vi "Calculate spot profile.vi"() -> ()   [LabVIEW 2012]
uses:
  <vilib>/Utility/file.llb/Write To Spreadsheet File (DBL).vi
panel:
  in  "Intensity":bool
  in  "log":bool
  in  "Save":bool
  in  "N spots":i32=2
  in  "xlog":dbl=2.0
  in  "stop 2":bool
  in  "Minimum":dbl(slide)=-3.5369774919614088 scale=-100.0..100.0
  in  "Maximum mult":dbl(slide)=0.9919614147909966 scale=0.1..2.0
  in  "stop":bool
  out "Spot profile":dbl[][](graph)
  out "Amplitudes/weights":sgl[][](graph)
  in  "I":sgl[](array[numeric])=[7.0, 7.0, 7.0, 7.0, 7.0, 7.0, 10.0, 10.0, 10.0, 10.0, 10.0, 10.0, 10.0, 10.0, 10.0, 10.0, 10.0, 10.0, 10.0, 10.0, 10.0]
  in  "xz-plane":bool=TRUE
  in  "step":sgl=1.0
  in  "N points":i32=512
  in  "Spot to display":i32
  in  "N_iterations":i32=100
  in  "x":sgl[](array[numeric])=[0.0, 40.0, -40.0, 10.0, 20.0, 30.0] format="%#_12g"
  in  "y":sgl[](array[numeric])=[0.0, 0.0, 0.0, 0.0, 0.0, 0.0, 0.0, 0.0, 0.0, 0.0, 0.0, 0.0, 0.0, 0.0, 0.0, 0.0, 0.0, 0.0, 0.0, 0.0, 0.0]
  in  "z":sgl[](array[numeric])=[0.0, 20.0, 20.0, -14.0, 0.0, 30.0, 0.0, 0.0, 0.0, 0.0, 0.0, 0.0, 0.0, 0.0, 0.0, 0.0, 0.0, 0.0, 0.0, 0.0, 0.0]
  in  "method":i32(ring)=1 items=["Lenses & gratings", "GS Fresnel", "GS FFT (2D)"]
  out "Generated Hologram":u8[][](graph)
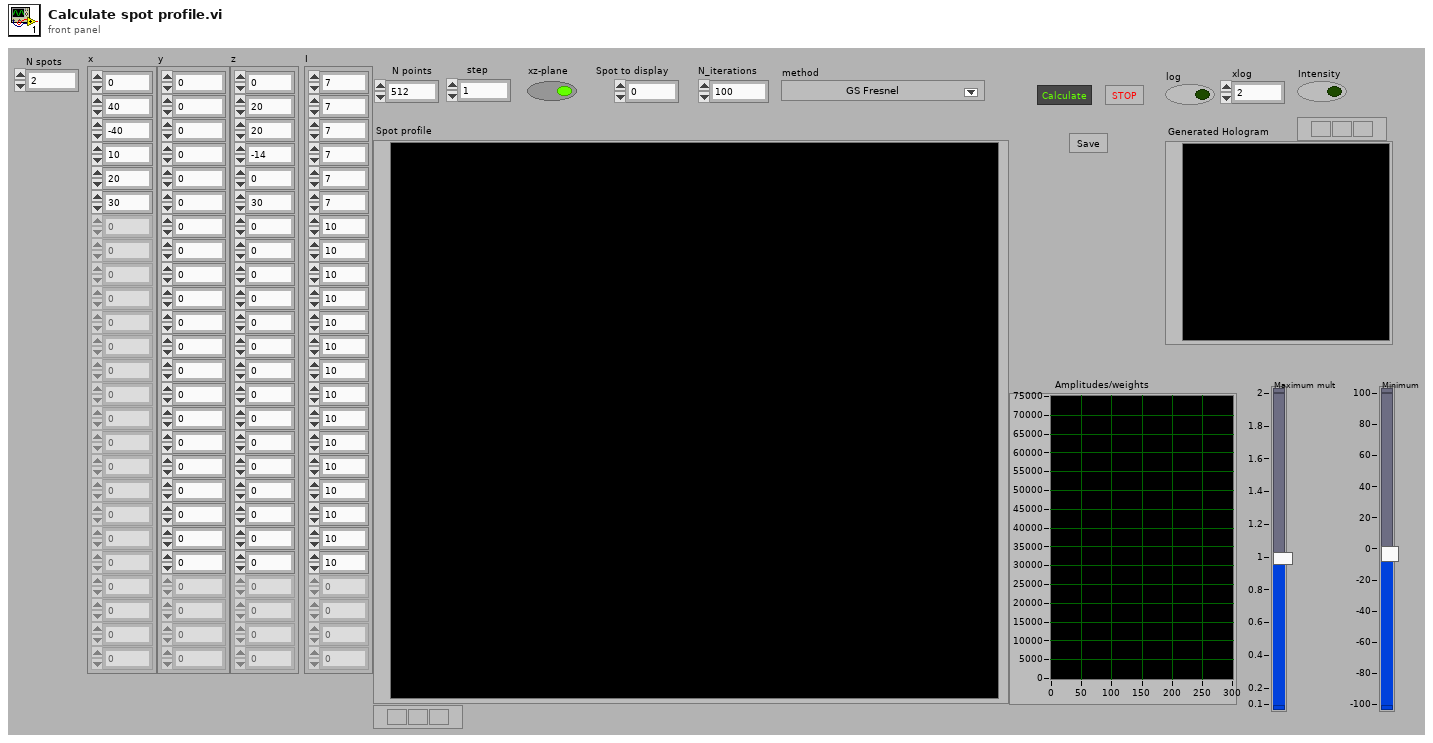
[diagram p1: front panel]
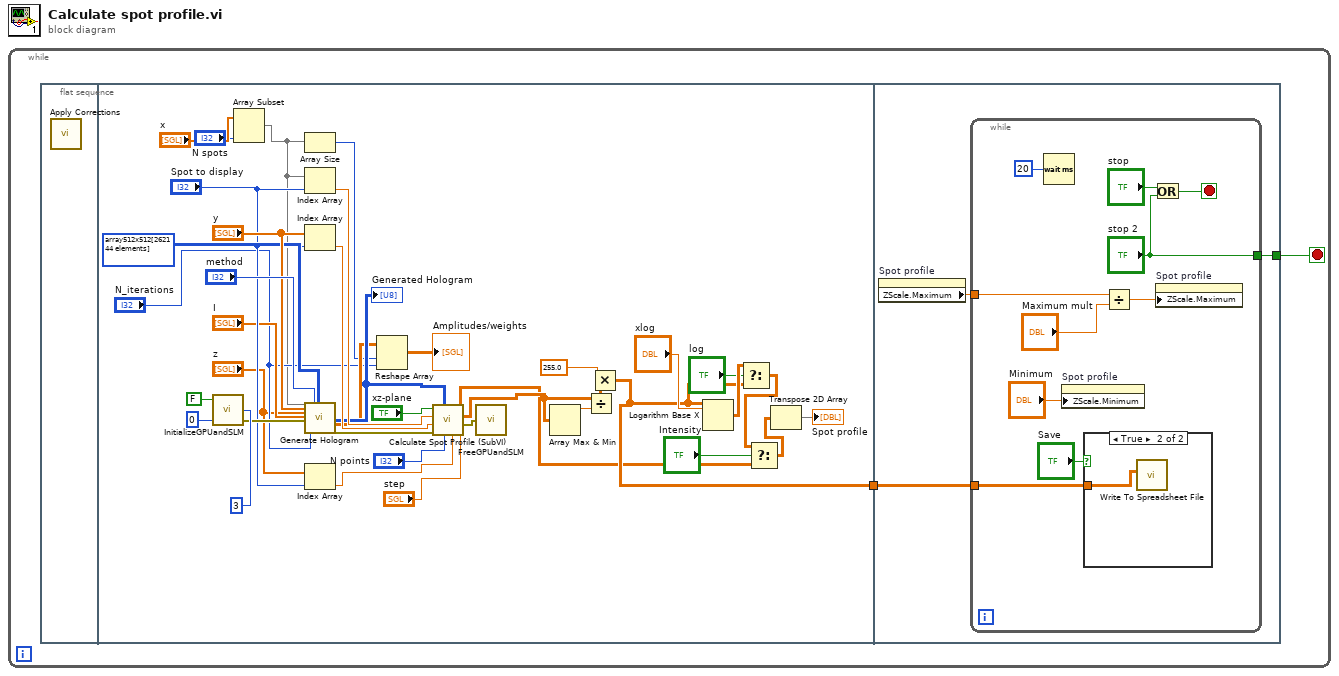
[diagram p0: block diagram]
diagram:
  n1 = while {
    stop <- w2 stop-if-true
    n2 = flat-sequence {
      tunnel: [w7] -> w1
      tunnel: [w43] -> w2
      tunnel: w1 -> [w42]
      frame #0 {
        n3 = call "Apply Corrections.vi"() -> ()  [unwired: 1 in]
      }
      frame #1 {
        n4 = call "InitializeGPUandSLM.vi"("TrueFrame"=3, "deviceId"=0 ("SLM size"), "SLM enabled"=FALSE) -> ("CUDA/SLM error"=w37:errorcluster)  [unwired: 1 in, 1 out]
        n5 = Array Subset(array="x", length="N spots") -> (w13:sgl[])  [unwired: 1 in]
        n6 = Array Size(array=w13) -> (size(s)=w22:i32)
        n7 = Index Array(array=w13, index="Spot to display") -> (element=w35:sgl)
        n8 = Index Array(array="y", index="Spot to display") -> (element=w34:sgl)
        n9 = call "Generate Hologram.vi"("x"=w13, "y"="y", "z"="z", "spot_intensities"="I", "CUDA/SLM error in"=w37, "N_iterations"="N_iterations", "method"="method", "CGH in"=u8[][] array512x512[262144 elements] ("Default")) -> ("CGH out"=w28:u8[][], "weights"=w23:sgl[][], "CUDA/SLM error out"=w29:errorcluster)  [unwired: 16 in, 1 out]
        "Generated Hologram" <- w28
        n10 = Index Array(array="z", index="Spot to display") -> (element=w32:sgl)
        n11 = Reshape Array(w23, w22, "N_iterations") -> (→"Amplitudes/weights":sgl[][])
        n12 = call "Calculate Spot Profile (SubVI).vi"("step"="step", "z"=w32, "N points"="N points", "CGH out"=w28, "CUDA/SLM error out"=w29, "y"=w34, "x"=w35, "xz-plane"="xz-plane") -> ("error out"=w30:errorcluster, "Calculated Intensity"=w12:sgl[][], "Calculated Phase"=w4:sgl[][])  [unwired: 1 out]
        n13 = call "FreeGPUandSLM.vi"("error in"=w30) -> ()  [unwired: 2 out]
        n14 = Array Max & Min(array=w12) -> (max value=w17:sgl)  [unwired: 3 out]
        n15 = Divide(x=w12, y=w17) -> (x/y=w9:sgl[][])
        n16 = Multiply(x=255.0 ("xlog"), y=w9) -> (x*y=w7:dbl[][])
        n17 = Logarithm Base X(1:"xlog", 2:w7) -> (0:w11:dbl[][])
        n18 = Select(t=w11, s="log", f=w7) -> (s? t:f=w6:dbl[][])
        n19 = Select(t=w6, s="Intensity", f=w4) -> (s? t:f=w5:dbl[][])
        n20 = Transpose 2D Array(2D array=w5) -> (transposed array=→"Spot profile":dbl[][])
      }
      frame #2 {
        n21 = property on="Spot profile" class="IntGraph (strict)"() -> ("ZScale.Maximum"=w44:dbl)  [unwired: 2 in, 2 out]
        n22 = while {
          tunnel: w44 -> [w53]
          tunnel: ["stop 2"] -> w43
          tunnel: w42 -> [w45]
          stop <- w48 stop-if-true
          n23 = Wait (ms)(milliseconds to wait=u32 20) -> ()  [unwired: 1 out]
          n24 = property on="Spot profile" class="IntGraph (strict)"("ZScale.Minimum"="Minimum") -> ()  [unwired: 2 in, 2 out]
          n25 = case shown="True" "Save" {
            tunnel: w45 -> [_ w55]
            frame False {
            }
            frame True {
              n26 = call-poly <vilib>:"Write To Spreadsheet File.vi"("2D data"=w55) -> ()  [unwired: 7 in, 1 out]
            }
          }
          n27 = Divide(x=w53, y="Maximum mult") -> (x/y=w51:dbl)
          n28 = Or(x="stop", y="stop 2") -> (x .or. y?=w48:bool)
          n29 = property on="Spot profile" class="IntGraph (strict)"("ZScale.Maximum"=w51) -> ()  [unwired: 2 in, 2 out]
        }
      }
    }
  }
